vi "UI Button Enable Disable_General.vi"(0 "Controls and Indicators\nReferences":T1, 1 "UI States":T7={"Inspection"={"Inspection States"=enum."Back _Inspection"}, "Diagnostics"={"Diagnostics States"=enum."Enable All"}, "Edit Tolerance"={"Edit Limits"=enum."Update List", "Enable Disable Measurements"=enum."Back to Edit Tolerance", "Page Select"=enum."Edit Tolerance Limits"}, "Page Select"=enum."Edit Tolerance"}, 3 "error in (no error)":errorcluster) -> (10 "error out":errorcluster)   [LabVIEW 2019, in "ZenGage v3.0 UI.lvclass"]
uses:
  ZenGage v3.0 UI.lvclass
  Type Definitions/General/UI States(UI button enable disable).ctl
  Type Definitions/Controls and Indicators/Select a part (combobox).ctl
  Type Definitions/Controls and Indicators/EDL control references.ctl
  Type Definitions/Controls and Indicators/Diagnostics control referencs.ctl
  Type Definitions/Controls and Indicators/Inspection control references.ctl
  Type Definitions/Controls and Indicators/General_Control references.ctl
  Type Definitions/Controls and Indicators/Controls and Indicators Cluster.ctl
  Type Definitions/General/Master sample references.ctl
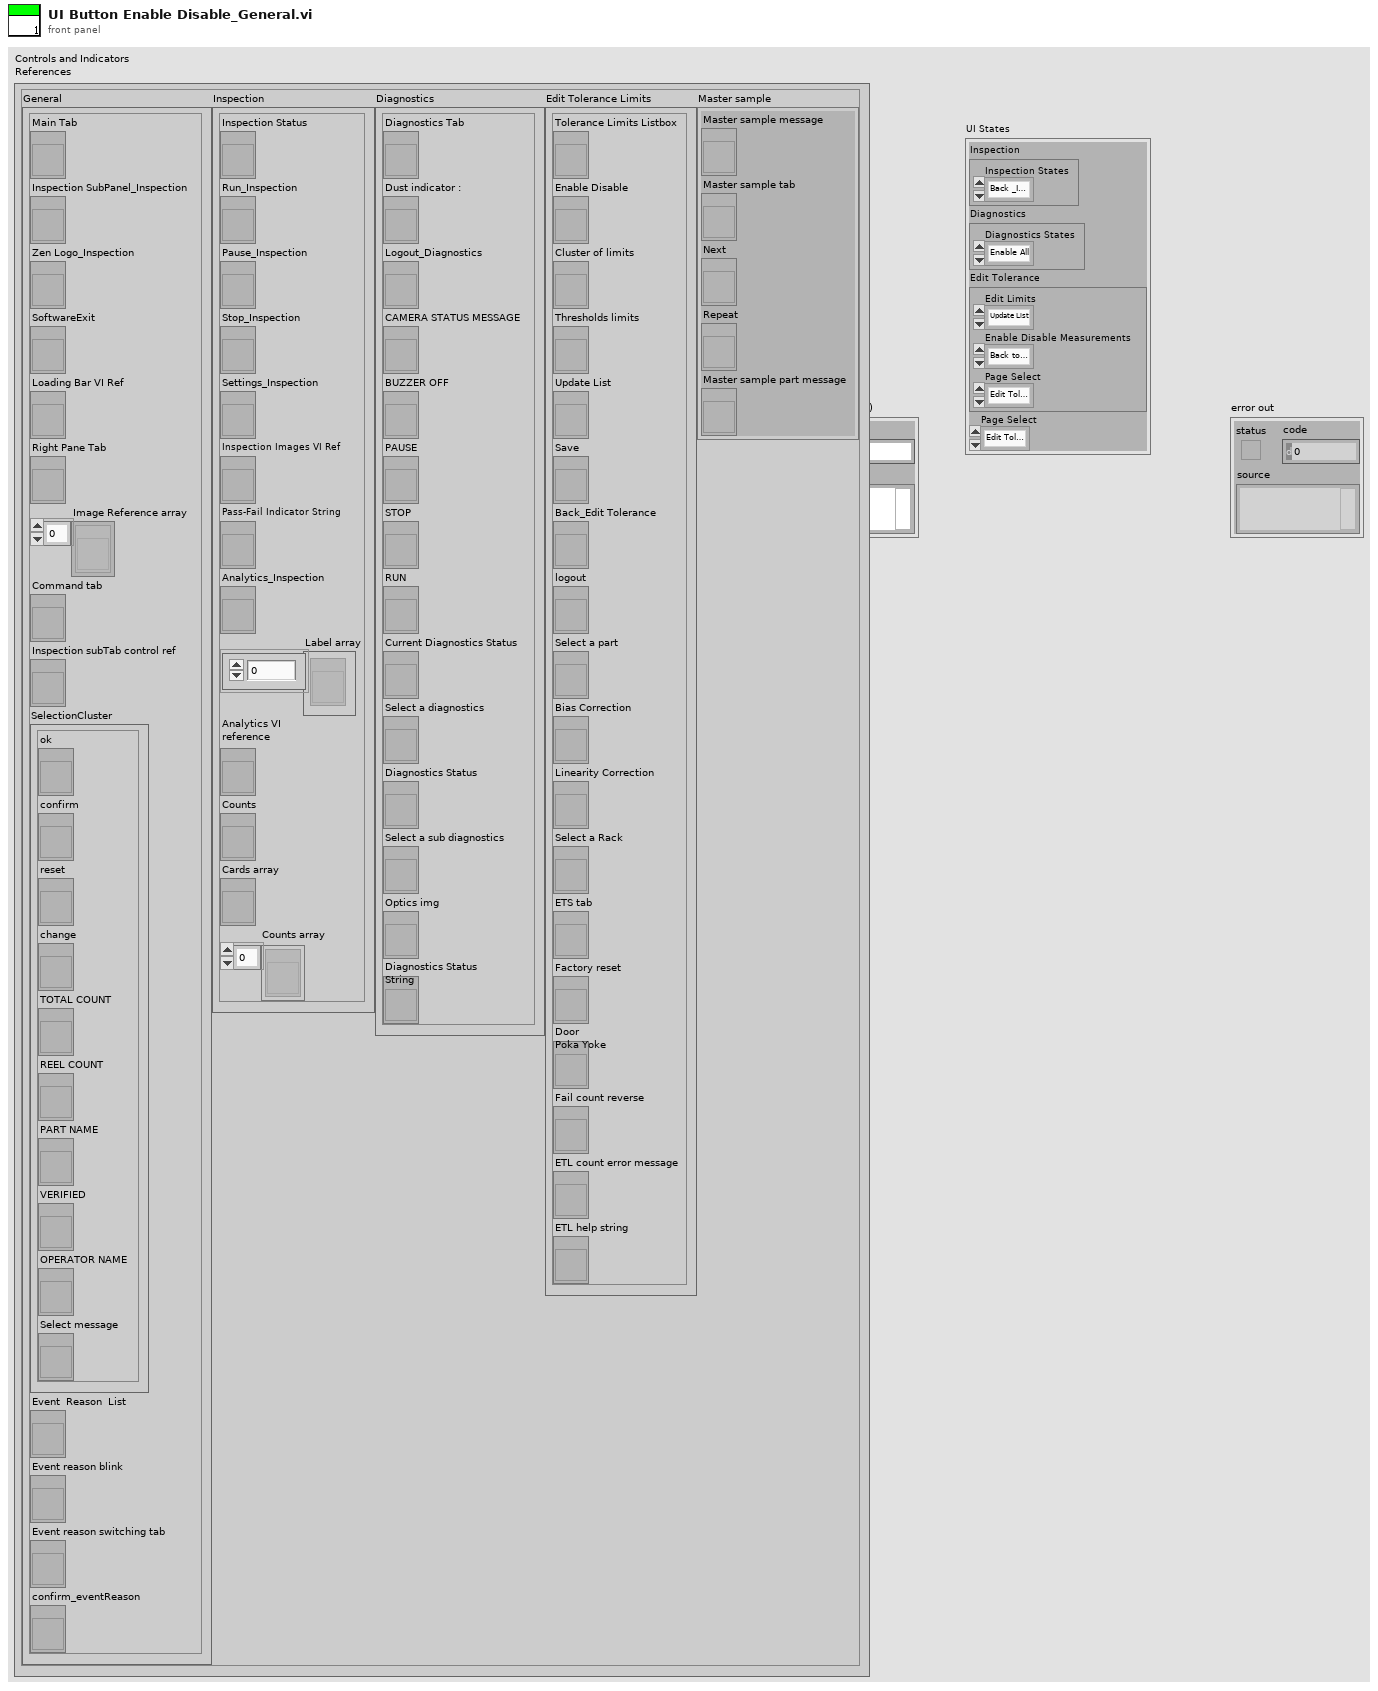
[diagram p1: front panel]
types:
  T1 = typedef "ZenGage v3.0 UI.lvclass/Controls and Indicators Cluster.ctl" = cluster{"General":T2, "Inspection":T3, "Diagnostics":T4, "Edit Tolerance Limits":T5, "Master sample":T6}
  T2 = typedef "ZenGage v3.0 UI.lvclass/General_Control references.ctl" = cluster{"Main Tab":refnum<vi>, "Inspection SubPanel_Inspection":refnum<vi>, "Zen Logo_Inspection":refnum<vi>, "SoftwareExit":refnum<vi>, "Loading Bar VI Ref":refnum<vi>, "Right Pane Tab":refnum<vi>, "Image Reference array":refnum<vi>[], "Command tab":refnum<vi>, "Inspection subTab control ref":refnum<vi>, "SelectionCluster":cluster{"ok":refnum<vi>, "confirm":refnum<vi>, "reset":refnum<vi>, "change":refnum<vi>, "TOTAL COUNT":refnum<vi>, "REEL COUNT":refnum<vi>, "PART NAME":refnum<vi>, "VERIFIED":refnum<vi>, "OPERATOR NAME":refnum<vi>, "Select message":refnum<vi>}, "Event  Reason  List":refnum<vi>, "Event reason blink":refnum<vi>, "Event reason switching tab":refnum<vi>, "confirm_eventReason":refnum<vi>}
  T3 = typedef "ZenGage v3.0 UI.lvclass/Inspection control references.ctl" = cluster{"Inspection Status":refnum<vi>, "Run_Inspection":refnum<vi>, "Pause_Inspection":refnum<vi>, "Stop_Inspection":refnum<vi>, "Settings_Inspection":refnum<vi>, "Inspection Images VI Ref":refnum<vi>, "Pass-Fail Indicator String":refnum<vi>, "Analytics_Inspection":refnum<vi>, "Label array":refnum<vi>[], "Analytics VI\nreference":refnum<vi>, "Counts":refnum<vi>, "Cards array":refnum<vi>, "Counts array":refnum<vi>[]}
  T4 = typedef "ZenGage v3.0 UI.lvclass/Diagnostics control referencs.ctl" = cluster{"Diagnostics Tab":refnum<vi>, "Dust indicator :":refnum<vi>, "Logout_Diagnostics":refnum<vi>, "CAMERA STATUS MESSAGE":refnum<vi>, "BUZZER OFF":refnum<vi>, "PAUSE":refnum<vi>, "STOP":refnum<vi>, "RUN":refnum<vi>, "Current Diagnostics Status":refnum<vi>, "Select a diagnostics":refnum<vi>, "Diagnostics Status":refnum<vi>, "Select a sub diagnostics":refnum<vi>, "Optics img":refnum<vi>, "Diagnostics Status\nString":refnum<vi>}
  T5 = typedef "ZenGage v3.0 UI.lvclass/EDL control references.ctl" = cluster{"Tolerance Limits Listbox":refnum<vi>, "Enable Disable":refnum<vi>, "Cluster of limits":refnum<vi>, "Thresholds limits":refnum<vi>, "Update List":refnum<vi>, "Save":refnum<vi>, "Back_Edit Tolerance":refnum<vi>, "logout":refnum<vi>, "Select a part":refnum<vi>, "Bias Correction":refnum<vi>, "Linearity Correction":refnum<vi>, "Select a Rack":refnum<vi>, "ETS tab":refnum<vi>, "Factory reset":refnum<vi>, "Door\nPoka Yoke":refnum<vi>, "Fail count reverse":refnum<vi>, "ETL count error message":refnum<vi>, "ETL help string":refnum<vi>}
  T6 = typedef "Master sample references.ctl" = cluster{"Master sample message":refnum<vi>, "Master sample tab":refnum<vi>, "Next":refnum<vi>, "Repeat":refnum<vi>, "Master sample part message":refnum<vi>}
  T7 = typedef "ZenGage v3.0 UI.lvclass/UI States(UI button enable disable).ctl" = cluster{"Inspection":cluster{"Inspection States":enum16{"PreSelect", "Back _Inspection", "Analytics", "Ready To Run", "Ready To Insert", "Enable All buttons", "Disable All Buttons", "Settings", "Select", "Stop", "Pause", "Inspect"}}, "Diagnostics":cluster{"Diagnostics States":enum16{"Enable All", "Camera Optics Fail", "Loading Bar", "Camera Optics", "Motor", "Arduino", "POST Done", "POST"}}, "Edit Tolerance":cluster{"Edit Limits":enum16{"Update List"}, "Enable Disable Measurements":enum16{"Back to Edit Tolerance"}, "Page Select":enum16{"Edit Tolerance Limits", "Enable Disable Buttons"}}, "Page Select":enum16{"Edit Tolerance", "Diagnostics", "Inspection"}}
  T8 = enum32{"Analytics", "Blank", "Diagnostics", "Run", "Edit Tolerance Settings"}
  T9 = enum32{"Inspection", "Diagnostics", "Edit Tolerance Settings"}
  T10 = enum32{"Edit Tolerance Limits1", "Inspection", "Master sample", "Diagnostics"}
  T11 = enum8{"Enabled", "Disabled", "Disabled and Grayed Out"}
  T12 = enum32{"Arduino Motor", "Sensor trigger", "Hardware Button", "Camera Optics"}
  T13 = enum16{"Edit Tolerance", "Diagnostics", "Inspection"}
  T14 = enum16{"Edit Tolerance Limits", "Enable Disable Buttons"}
  T15 = enum16{"Enable All", "Camera Optics Fail", "Loading Bar", "Camera Optics", "Motor", "Arduino", "POST Done", "POST"}
  T16 = enum16{"PreSelect", "Back _Inspection", "Analytics", "Ready To Run", "Ready To Insert", "Enable All buttons", "Disable All Buttons", "Settings", "Select", "Stop", "Pause", "Inspect"}
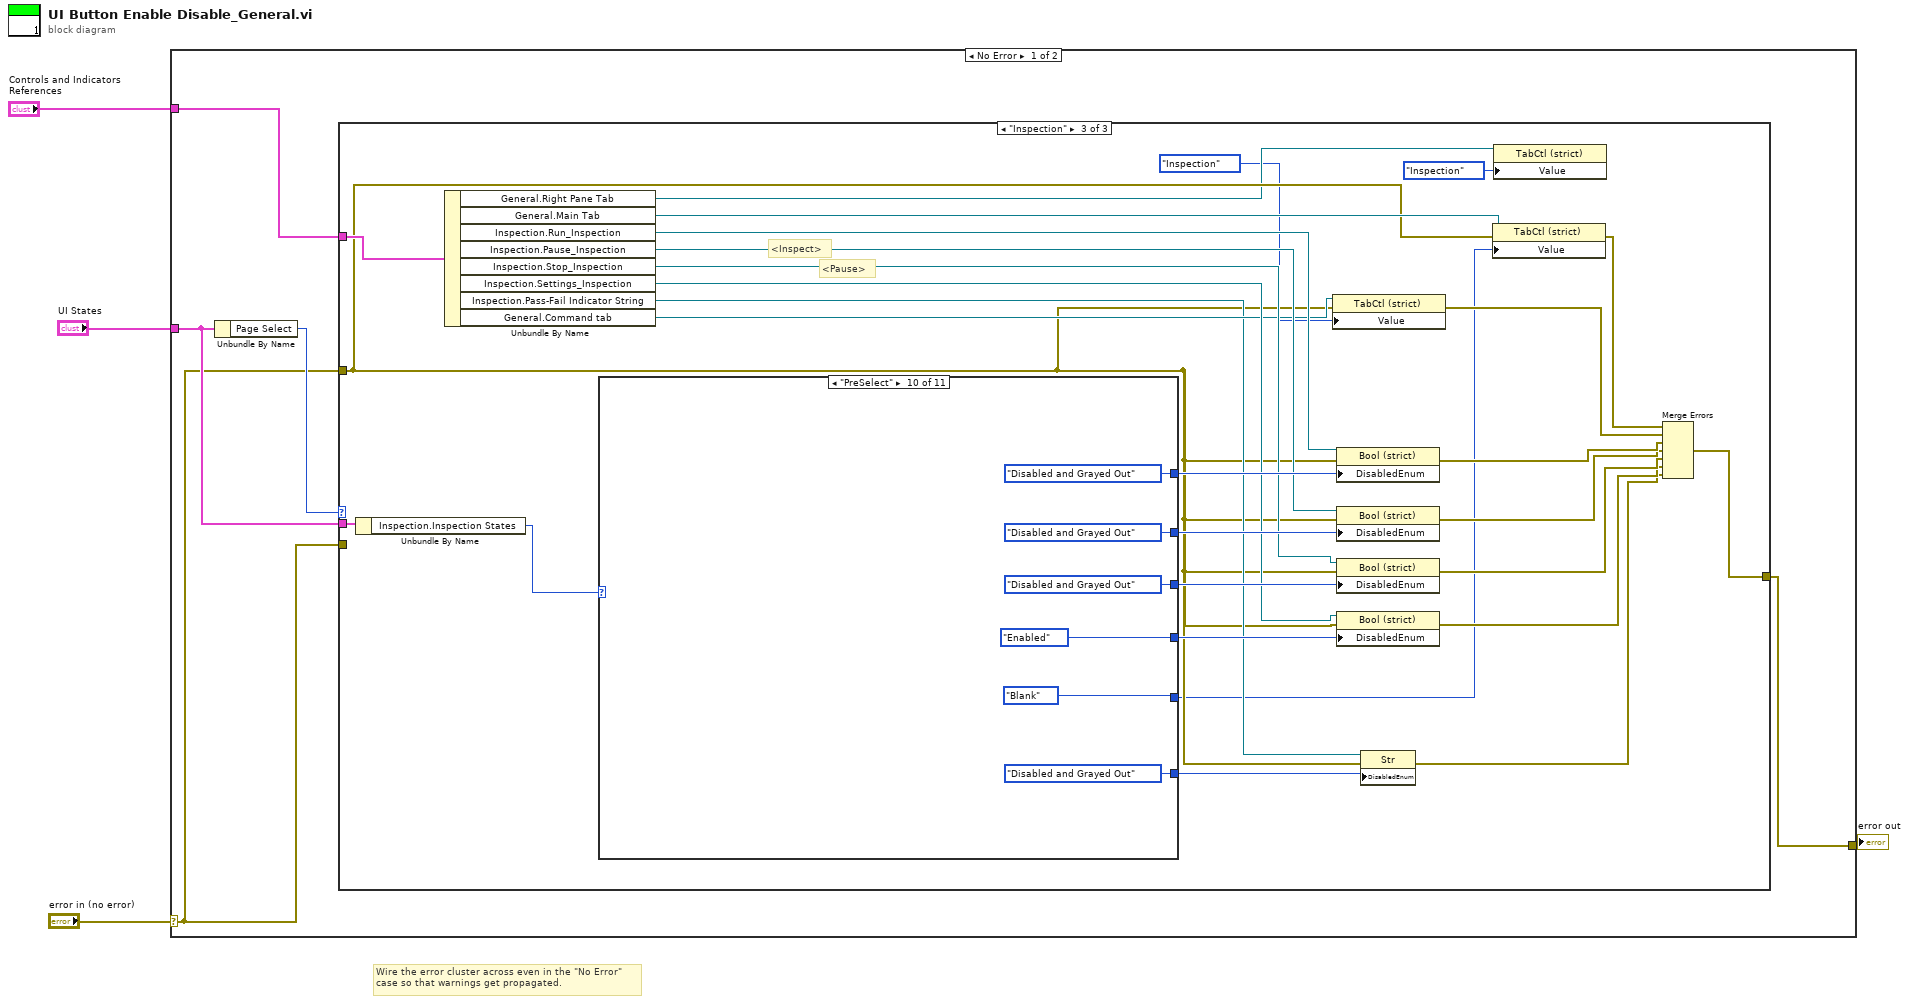
[diagram p0: block diagram]
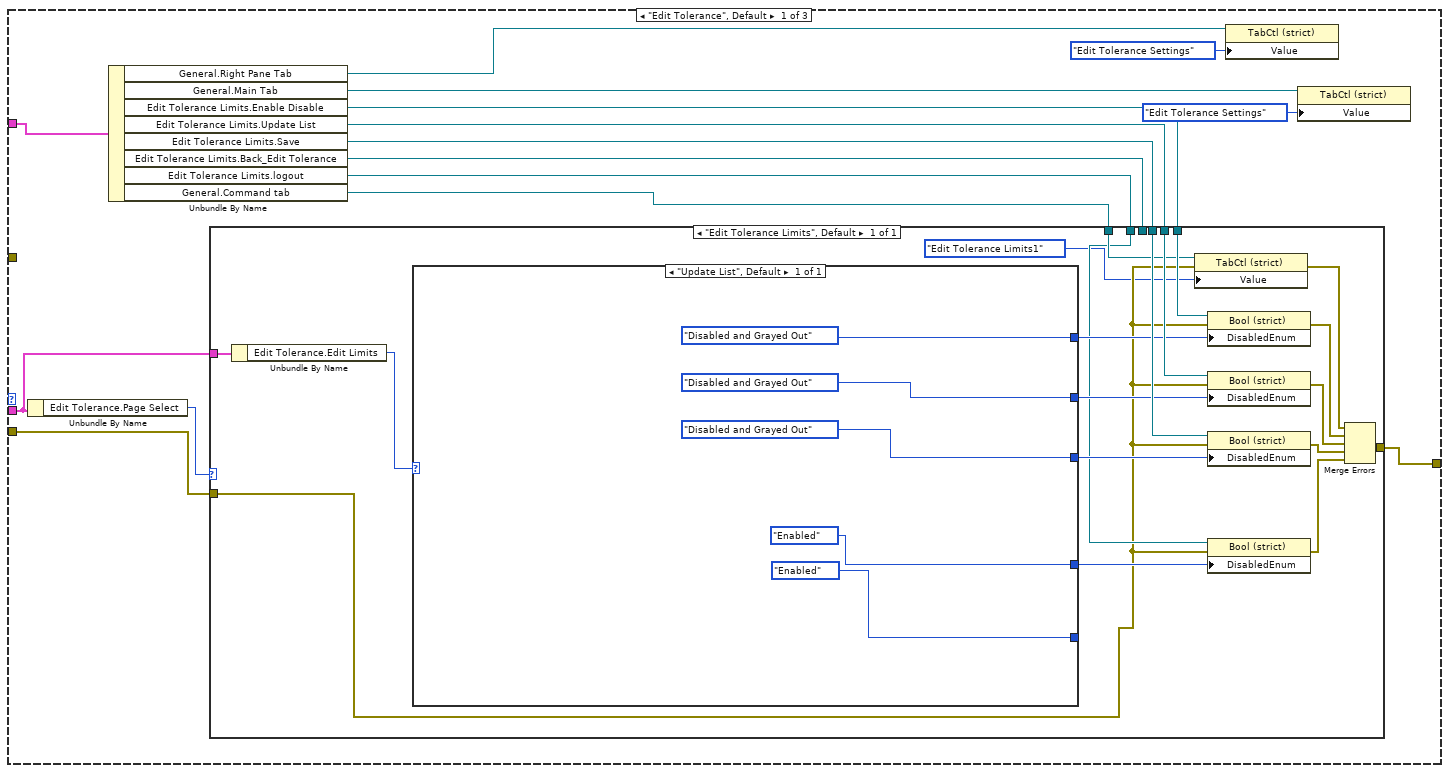
[diagram p2: hidden frame]
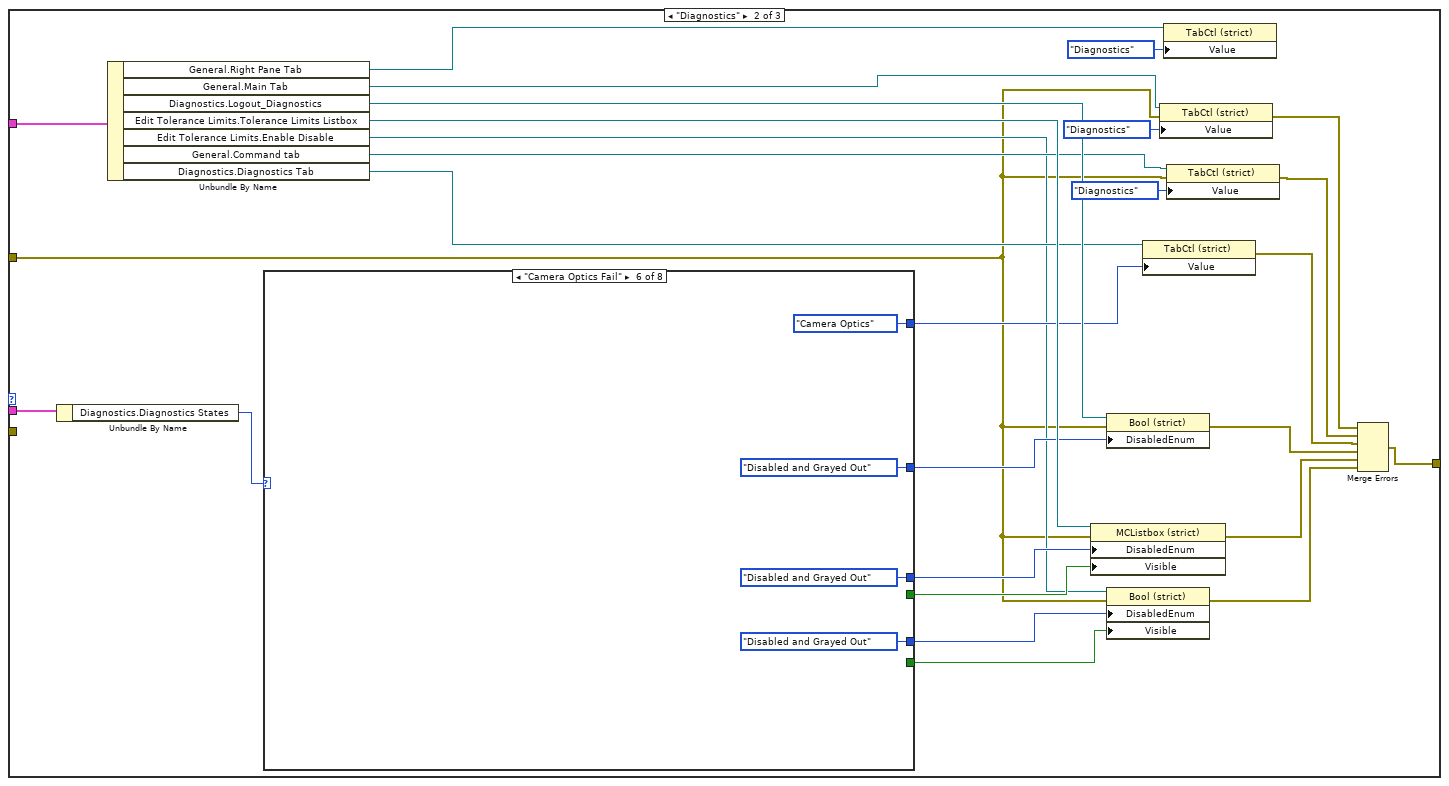
[diagram p3: hidden frame]
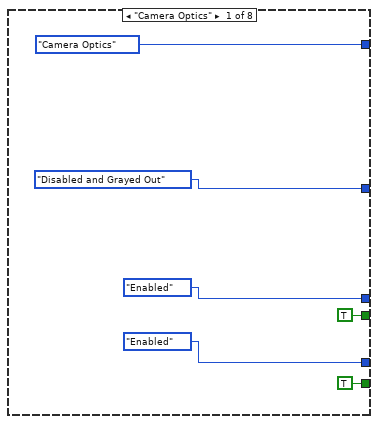
[diagram p4: hidden frame]
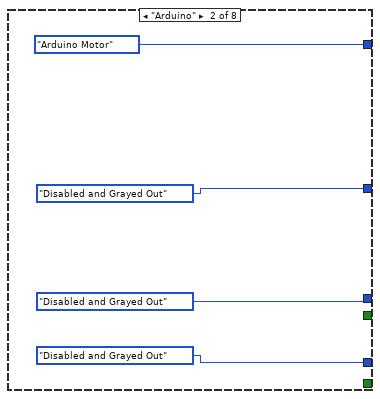
[diagram p5: hidden frame]
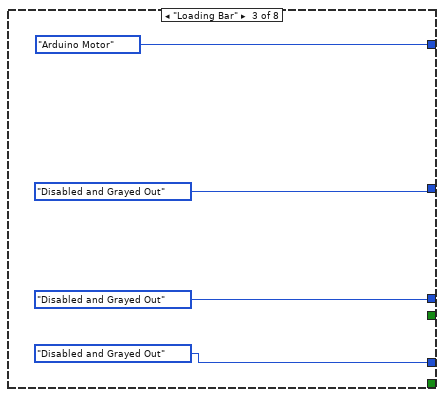
[diagram p6: hidden frame]
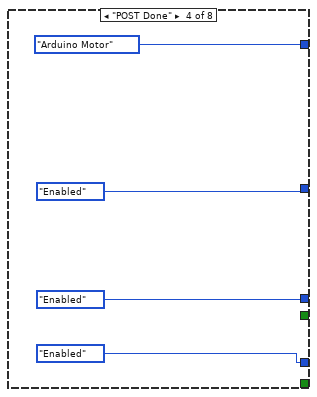
[diagram p7: hidden frame]
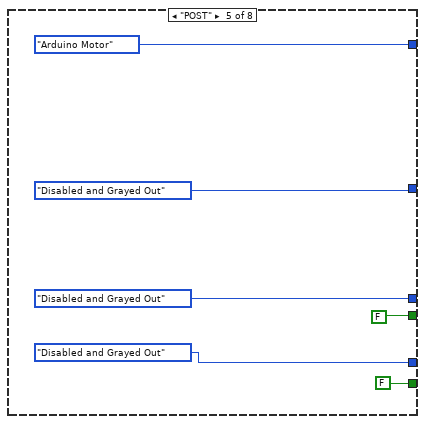
[diagram p8: hidden frame]
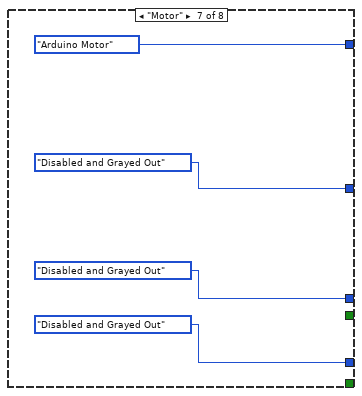
[diagram p9: hidden frame]
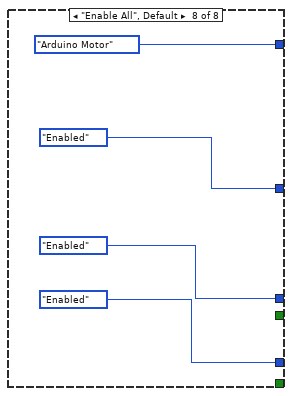
[diagram p10: hidden frame]
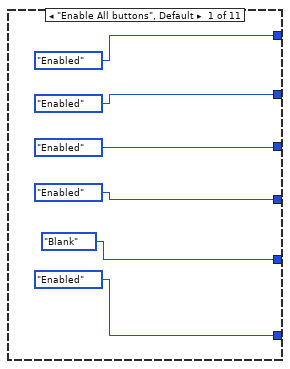
[diagram p11: hidden frame]
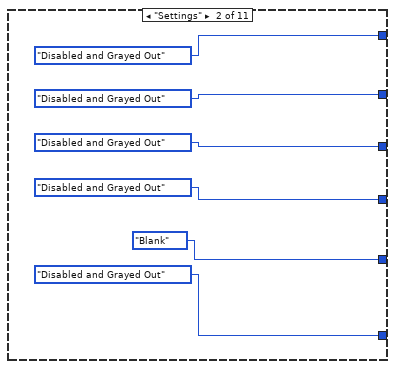
[diagram p12: hidden frame]
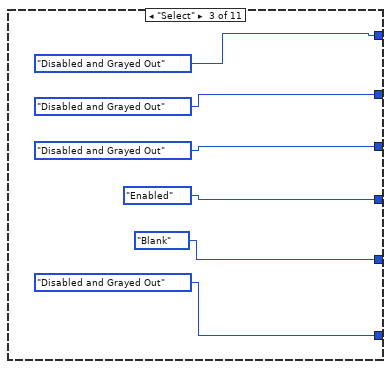
[diagram p13: hidden frame]
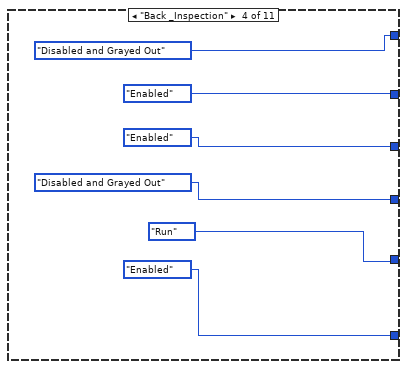
[diagram p14: hidden frame]
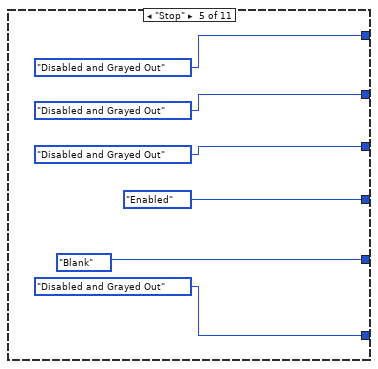
[diagram p15: hidden frame]
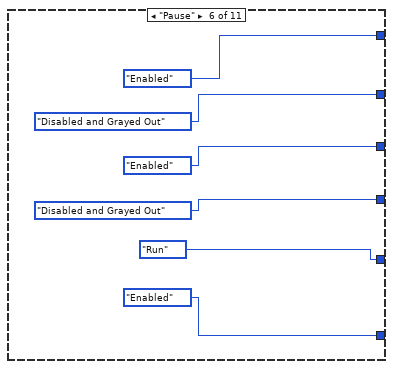
[diagram p16: hidden frame]
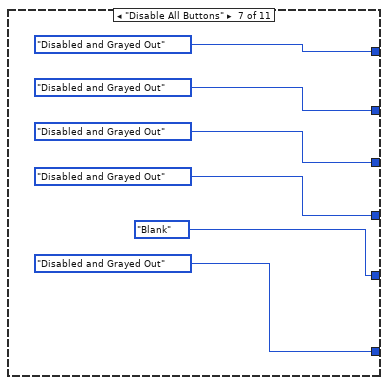
[diagram p17: hidden frame]
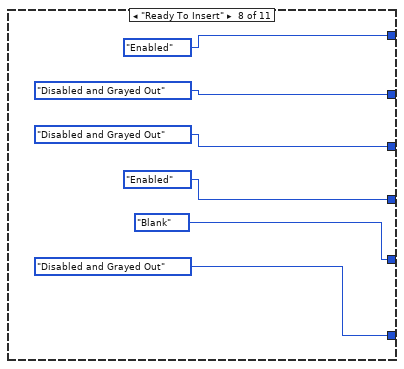
[diagram p18: hidden frame]
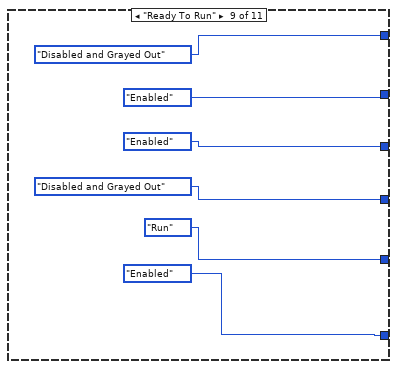
[diagram p19: hidden frame]
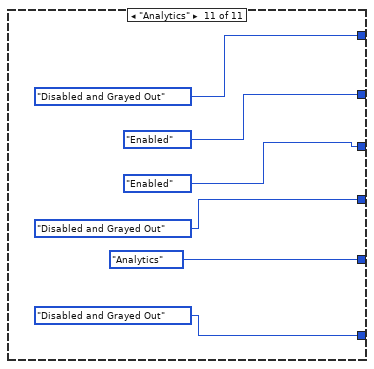
[diagram p20: hidden frame]
diagram:
  # "Wire the error cluster across even in the \"No Error\"\ncase so that warnings get propagated."
  n1 = case shown="No Error" "error in (no error)" {
    selector: "error in (no error)" -> [w6 w206]
    tunnel: "Controls and Indicators\nReferences" -> [w8 _]
    tunnel: "UI States" -> [w7 _]
    tunnel: [w5 w206] -> w2
    frame No Error {
      n2 = Unbundle By Name(w7) -> ("Page Select"=w9:T13)
      n3 = case shown="\"Inspection\"" w9 {
        tunnel: w8 -> [w24 w75 w139]
        tunnel: w7 -> [w22 w74 w138]
        tunnel: w6 -> [_ w49 w124]
        tunnel: [w13 w56 w116] -> w5
        tunnel: w6 -> [w14 _ _]
        frame "Edit Tolerance", Default {
          n4 = Unbundle By Name(w22) -> ("Edit Tolerance.Page Select"=w23:T14)
          n5 = Unbundle By Name(w24) -> ("General.Right Pane Tab"=w12:refnum<vi>, "General.Main Tab"=w16:refnum<vi>, "Edit Tolerance Limits.Enable Disable"=w17:refnum<vi>, "Edit Tolerance Limits.Update List"=w21:refnum<vi>, "Edit Tolerance Limits.Save"=w20:refnum<vi>, "Edit Tolerance Limits.Back_Edit Tolerance"=w19:refnum<vi>, "Edit Tolerance Limits.logout"=w18:refnum<vi>, "General.Command tab"=w15:refnum<vi>)
          n6 = case shown="\"Edit Tolerance Limits\", Default" w23 {
            tunnel: w22 -> [w43]
            tunnel: w21 -> [w40]
            tunnel: w20 -> [w39]
            tunnel: w19 -> [_]
            tunnel: w18 -> [w29]
            tunnel: w17 -> [w41]
            tunnel: w15 -> [w35]
            tunnel: w14 -> [w26]
            tunnel: [w30] -> w13
            frame "Edit Tolerance Limits", Default {
              n7 = Unbundle By Name(w43) -> ("Edit Tolerance.Edit Limits"=w42:enum16{"Update List"})
              n8 = case shown="\"Update List\", Default" w42 {
                tunnel: [T11."Disabled and Grayed Out" ("Disabled")] -> w38
                tunnel: [T11."Disabled and Grayed Out" ("Disabled")] -> w37
                tunnel: [T11."Disabled and Grayed Out" ("Disabled")] -> w36
                tunnel: [T11."Enabled" ("Disabled")] -> _
                tunnel: [T11."Enabled" ("Disabled")] -> w28
                frame "Update List", Default {
                }
              }
              n9 = property class="TabCtl (strict)"(reference=w35, error in=w26, "Value"=T10."Edit Tolerance Limits1") -> (error out=w34:errorcluster)  [unwired: 1 out]
              n10 = property class="Bool (strict)"(reference=w41, error in=w26, "DisabledEnum"=w38) -> (error out=w33:errorcluster)  [unwired: 1 out]
              n11 = property class="Bool (strict)"(reference=w40, error in=w26, "DisabledEnum"=w37) -> (error out=w32:errorcluster)  [unwired: 1 out]
              n12 = property class="Bool (strict)"(reference=w39, error in=w26, "DisabledEnum"=w36) -> (error out=w31:errorcluster)  [unwired: 1 out]
              n13 = property class="Bool (strict)"(reference=w29, error in=w26, "DisabledEnum"=w28) -> (error out=w27:errorcluster)  [unwired: 1 out]
              n14 = Merge Errors(w34, w33, w32, w31, w27) -> (w30:errorcluster)
            }
          }
          n15 = property class="TabCtl (strict)"(reference=w12, "Value"=T9."Edit Tolerance Settings") -> ()  [unwired: 1 in, 2 out]
          n16 = property class="TabCtl (strict)"(reference=w16, "Value"=T8."Edit Tolerance Settings") -> ()  [unwired: 1 in, 2 out]
        }
        frame "Diagnostics" {
          n17 = Unbundle By Name(w74) -> ("Diagnostics.Diagnostics States"=w73:T15)
          n18 = Unbundle By Name(w75) -> ("General.Right Pane Tab"=w54:refnum<vi>, "General.Main Tab"=w67:refnum<vi>, "Diagnostics.Logout_Diagnostics"=w72:refnum<vi>, "Edit Tolerance Limits.Tolerance Limits Listbox"=w71:refnum<vi>, "Edit Tolerance Limits.Enable Disable"=w51:refnum<vi>, "General.Command tab"=w64:refnum<vi>, "Diagnostics.Diagnostics Tab"=w63:refnum<vi>)
          n19 = case shown="\"Camera Optics Fail\"" w73 {
            tunnel: [T11."Disabled and Grayed Out" ("Disabled") T11."Disabled and Grayed Out" ("Disabled") T11."Disabled and Grayed Out" ("Disabled") T11."Enabled" ("Disabled") T11."Disabled and Grayed Out" ("Disabled") T11."Disabled and Grayed Out" ("Disabled") T11."Disabled and Grayed Out" ("Disabled") T11."Enabled" ("Disabled")] -> w70
            tunnel: [T11."Enabled" ("Disabled") T11."Disabled and Grayed Out" ("Disabled") T11."Disabled and Grayed Out" ("Disabled") T11."Enabled" ("Disabled") T11."Disabled and Grayed Out" ("Disabled") T11."Disabled and Grayed Out" ("Disabled") T11."Disabled and Grayed Out" ("Disabled") T11."Enabled" ("Disabled")] -> w69
            tunnel: [T11."Enabled" ("Disabled") T11."Disabled and Grayed Out" ("Disabled") T11."Disabled and Grayed Out" ("Disabled") T11."Enabled" ("Disabled") T11."Disabled and Grayed Out" ("Disabled") T11."Disabled and Grayed Out" ("Disabled") T11."Disabled and Grayed Out" ("Disabled") T11."Enabled" ("Disabled")] -> w68
            tunnel: [TRUE ("Visible") _ _ _ FALSE ("Visible") _ _ _] -> w66
            tunnel: [TRUE ("Visible") _ _ _ FALSE ("Visible") _ _ _] -> w65
            tunnel: [T12."Camera Optics" ("Value") T12."Arduino Motor" ("Value") T12."Arduino Motor" ("Value") T12."Arduino Motor" ("Value") T12."Arduino Motor" ("Value") T12."Camera Optics" ("Value") T12."Arduino Motor" ("Value") T12."Arduino Motor" ("Value")] -> w52
            frame "Camera Optics" {
            }
            frame "Arduino" {
            }
            frame "Loading Bar" {
            }
            frame "POST Done" {
            }
            frame "POST" {
            }
            frame "Camera Optics Fail" {
            }
            frame "Motor" {
            }
            frame "Enable All", Default {
            }
          }
          n20 = property class="MCListbox (strict)"(reference=w71, error in=w49, "DisabledEnum"=w69, "Visible"=w66) -> (error out=w58:errorcluster)  [unwired: 1 out]
          n21 = property class="Bool (strict)"(reference=w72, error in=w49, "DisabledEnum"=w70) -> (error out=w59:errorcluster)  [unwired: 1 out]
          n22 = property class="Bool (strict)"(reference=w51, error in=w49, "DisabledEnum"=w68, "Visible"=w65) -> (error out=w57:errorcluster)  [unwired: 1 out]
          n23 = property class="TabCtl (strict)"(reference=w63, "Value"=w52) -> (error out=w60:errorcluster)  [unwired: 1 in, 1 out]
          n24 = property class="TabCtl (strict)"(reference=w67, error in=w49, "Value"=T8."Diagnostics") -> (error out=w62:errorcluster)  [unwired: 1 out]
          n25 = property class="TabCtl (strict)"(reference=w54, "Value"=T9."Diagnostics") -> ()  [unwired: 1 in, 2 out]
          n26 = property class="TabCtl (strict)"(reference=w64, error in=w49, "Value"=T10."Diagnostics") -> (error out=w61:errorcluster)  [unwired: 1 out]
          n27 = Merge Errors(w62, w61, w60, w59, w58, w57) -> (w56:errorcluster)
        }
        frame "Inspection" {
          # "<Pause>"
          # "<Inspect>"
          n28 = Unbundle By Name(w138) -> ("Inspection.Inspection States"=w137:T16)
          n29 = Unbundle By Name(w139) -> ("General.Right Pane Tab"=w114:refnum<vi>, "General.Main Tab"=w127:refnum<vi>, "Inspection.Run_Inspection"=w131:refnum<vi>, "Inspection.Pause_Inspection"=w130:refnum<vi>, "Inspection.Stop_Inspection"=w129:refnum<vi>, "Inspection.Settings_Inspection"=w128:refnum<vi>, "Inspection.Pass-Fail Indicator String"=w125:refnum<vi>, "General.Command tab"=w126:refnum<vi>)
          n30 = case shown="\"PreSelect\"" w137 {
            tunnel: [T11."Enabled" ("Disabled") T11."Disabled and Grayed Out" ("Disabled") T11."Disabled and Grayed Out" ("Disabled") T11."Disabled and Grayed Out" ("Disabled") T11."Disabled and Grayed Out" ("Disabled") T11."Enabled" ("Disabled") T11."Disabled and Grayed Out" ("Disabled") T11."Enabled" ("Disabled") T11."Disabled and Grayed Out" ("Disabled") T11."Disabled and Grayed Out" ("Disabled") T11."Disabled and Grayed Out" ("Disabled")] -> w136
            tunnel: [T11."Enabled" ("Disabled") T11."Disabled and Grayed Out" ("Disabled") T11."Disabled and Grayed Out" ("Disabled") T11."Enabled" ("Disabled") T11."Disabled and Grayed Out" ("Disabled") T11."Disabled and Grayed Out" ("Disabled") T11."Disabled and Grayed Out" ("Disabled") T11."Disabled and Grayed Out" ("Disabled") T11."Enabled" ("Disabled") T11."Disabled and Grayed Out" ("Disabled") T11."Enabled" ("Disabled")] -> w135
            tunnel: [T11."Enabled" ("Disabled") T11."Disabled and Grayed Out" ("Disabled") T11."Disabled and Grayed Out" ("Disabled") T11."Enabled" ("Disabled") T11."Disabled and Grayed Out" ("Disabled") T11."Enabled" ("Disabled") T11."Disabled and Grayed Out" ("Disabled") T11."Disabled and Grayed Out" ("Disabled") T11."Enabled" ("Disabled") T11."Disabled and Grayed Out" ("Disabled") T11."Enabled" ("Disabled")] -> w134
            tunnel: [T11."Enabled" ("Disabled") T11."Disabled and Grayed Out" ("Disabled") T11."Enabled" ("Disabled") T11."Disabled and Grayed Out" ("Disabled") T11."Enabled" ("Disabled") T11."Disabled and Grayed Out" ("Disabled") T11."Disabled and Grayed Out" ("Disabled") T11."Enabled" ("Disabled") T11."Disabled and Grayed Out" ("Disabled") T11."Enabled" ("Disabled") T11."Disabled and Grayed Out" ("Disabled")] -> w133
            tunnel: [T11."Enabled" ("Disabled") T11."Disabled and Grayed Out" ("Disabled") T11."Disabled and Grayed Out" ("Disabled") T11."Enabled" ("Disabled") T11."Disabled and Grayed Out" ("Disabled") T11."Enabled" ("Disabled") T11."Disabled and Grayed Out" ("Disabled") T11."Disabled and Grayed Out" ("Disabled") T11."Enabled" ("Disabled") T11."Disabled and Grayed Out" ("Disabled") T11."Disabled and Grayed Out" ("Disabled")] -> w132
            tunnel: [T8."Blank" ("Value") T8."Blank" ("Value") T8."Blank" ("Value") T8."Run" ("Value") T8."Blank" ("Value") T8."Run" ("Value") T8."Blank" ("Value") T8."Blank" ("Value") T8."Run" ("Value") T8."Blank" ("Value") T8."Analytics" ("Value")] -> w113
            frame "Enable All buttons", Default {
            }
            frame "Settings" {
            }
            frame "Select" {
            }
            frame "Back _Inspection" {
            }
            frame "Stop" {
            }
            frame "Pause" {
            }
            frame "Disable All Buttons" {
            }
            frame "Ready To Insert" {
            }
            frame "Ready To Run" {
            }
            frame "PreSelect" {
            }
            frame "Analytics" {
            }
          }
          n31 = property class="TabCtl (strict)"(reference=w126, error in=w124, "Value"=T10."Inspection") -> (error out=w122:errorcluster)  [unwired: 1 out]
          n32 = property class="Bool (strict)"(reference=w131, error in=w124, "DisabledEnum"=w136) -> (error out=w121:errorcluster)  [unwired: 1 out]
          n33 = property class="Bool (strict)"(reference=w130, error in=w124, "DisabledEnum"=w135) -> (error out=w120:errorcluster)  [unwired: 1 out]
          n34 = property class="Bool (strict)"(reference=w129, error in=w124, "DisabledEnum"=w134) -> (error out=w119:errorcluster)  [unwired: 1 out]
          n35 = property class="Bool (strict)"(reference=w128, error in=w124, "DisabledEnum"=w133) -> (error out=w118:errorcluster)  [unwired: 1 out]
          n36 = property class="Str"(reference=w125, error in=w124, "DisabledEnum"=w132) -> (error out=w117:errorcluster)  [unwired: 1 out]
          n37 = property class="TabCtl (strict)"(reference=w127, error in=w124, "Value"=w113) -> (error out=w123:errorcluster)  [unwired: 1 out]
          n38 = property class="TabCtl (strict)"(reference=w114, "Value"=T9."Inspection") -> ()  [unwired: 1 in, 2 out]
          n39 = Merge Errors(w123, w122, w121, w120, w119, w118, w117) -> (w116:errorcluster)
        }
      }
    }
    frame Error {
    }
  }
  "error out" <- w2
